vi "isInitialized.vi"(8 "error in (no error)":errorcluster, 11 "NotifierStopMechanism in":refnum<class "BoolNotifierStopMechanism.lvclass">) -> (0 "error out":errorcluster, 2 "isInitRequired":bool, 3 "NotifierStopMechanism out":refnum<class "BoolNotifierStopMechanism.lvclass">)   [LabVIEW 2023, in "TLC_Daemon.lvlib" / "BoolNotifierStopMechanism.lvclass"]
doc: "Returns True if the StopMechanism requires initialization.\nThis is useful for handling both of the following cases:\n- Internal Initialization: The StopMechanism is initialized by the TaskController, which handles the entire lifecycle.\n- External Initialization: The StopMechanism is already initialized externally. This is used when you need to share the mechanism with other components (such as message queues).\n\nNote: Use external initialization carefully; the TaskController sends stopRequests, which may impact external code.\n_____________________________________\nTLC Daemon 1.0.0.2\nCopyright (c) 2026 Andrea Cadei"
uses:
  BoolNotifierStopMech/BoolNotifierStopMechanism.lvclass
  BoolNotifierStopMech/BoolNotifierStopMechanism.lvclass/BoolNotifierStopMechanism.ctl
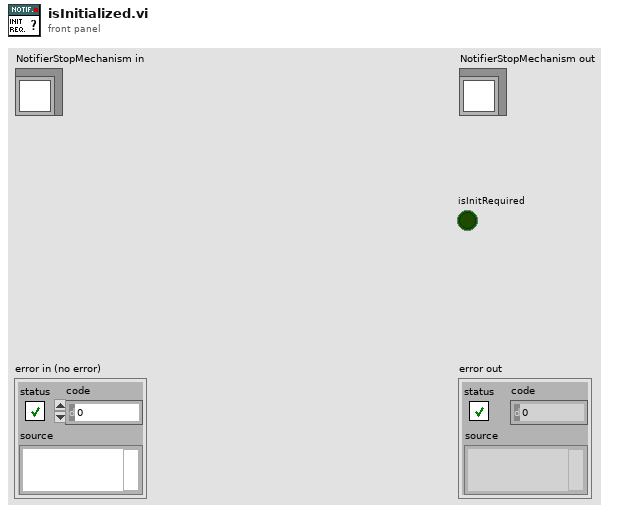
[diagram p1: front panel]
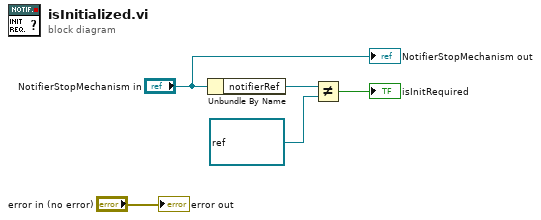
[diagram p0: block diagram]
diagram:
  n1 = Unbundle By Name("NotifierStopMechanism in") -> ("notifierRef"=w3:refnum<notifier>)
  n2 = Not Equal?(x=w3, y=refnum<notifier> refnum) -> (x != y?=→"isInitRequired":bool)
  "error out" <- "error in (no error)"
  "NotifierStopMechanism out" <- "NotifierStopMechanism in"
